vi "Parse.vi"(8 "error in (no error)":errorcluster, 10 "Data String":string, 11 "No-op Parser in":refnum<class "No-op Parser.lvclass">) -> (0 "error out":errorcluster, 2 "Data Values":dbl[](array[numeric]), 3 "No-op Parser out":refnum<class "No-op Parser.lvclass">)   [LabVIEW 2018, in "No-op Parser.lvclass"]
doc: "No-op Parser.lvclass:Parse.vi\n\nThis is the Parsing VI for the No-op Parser class. It creates an array of doubles from a string by unflattening it.\n\nInstrument Communication Module Version 1.0\nJanuary, 2018 Original Code Consulting David Thomson\n www.originalcode.com"
uses:
  No-op Parser.lvclass
  No-op Parser.lvclass/No-op Parser.ctl
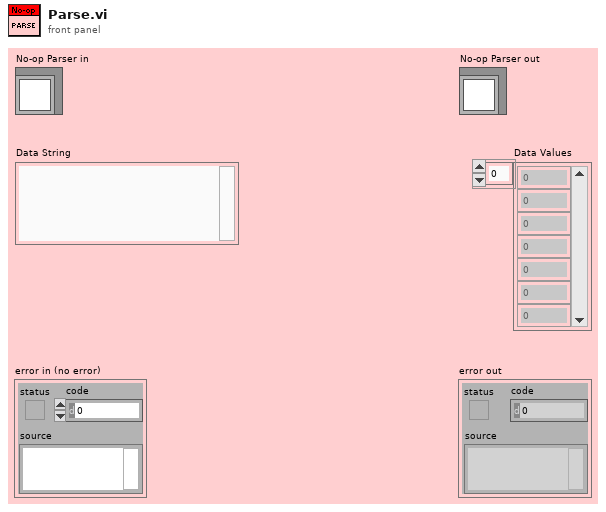
[diagram p1: front panel]
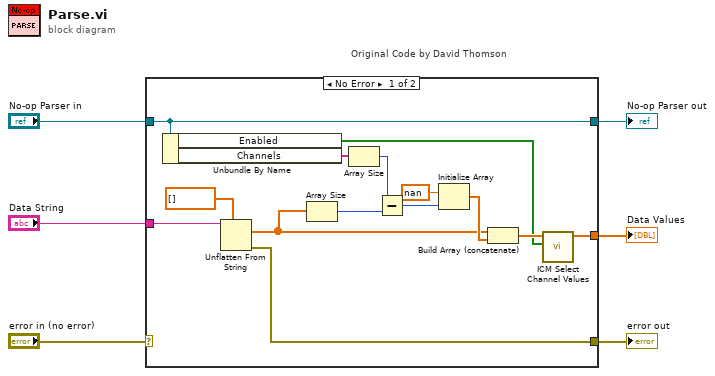
[diagram p0: block diagram]
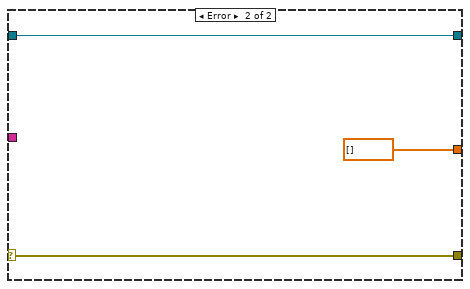
[diagram p2: hidden frame]
diagram:
  n1 = case "Original Code by David Thomson" shown="No Error" "error in (no error)" {
    selector: "error in (no error)" -> [_ w23]
    tunnel: "No-op Parser in" -> [w10 w22]
    tunnel: [w18 w23] -> w4
    tunnel: [w10 w22] -> w3
    tunnel: "Data String" -> [w20 _]
    tunnel: [w12 dbl[] []] -> w1
    frame No Error {
      n2 = Unbundle By Name(w10) -> ("Enabled"=w7:bool[], "Channels"=w9:string[])
      n3 = Unflatten From String(type=dbl[] [], binary string=w20) -> (value=w11:dbl[], error out=w18:errorcluster)  [unwired: 3 in, 1 out]
      n4 = Array Size(array=w11) -> (size(s)=w16:i32)
      n5 = Array Size(array=w9) -> (size(s)=w8:i32)
      n6 = Subtract(x=w8, y=w16) -> (x-y=w15:i32)
      n7 = Initialize Array(nan ("y"), w15) -> (w14:dbl[])
      n8 = Build Array (concatenate)(w11, w14) -> (w13:dbl[])
      n9 = call "ICM Select Channel Values.vi"("Enabled"=w7, "Channel Values"=w13) -> ("Enabled Values"=w12:dbl[])  [unwired: 9 in]
    }
    frame Error {
    }
  }
  "error out" <- w4
  "No-op Parser out" <- w3
  "Data Values" <- w1
